vi "Open Backpressure Reader.vi"(8 "error in (no error)":errorcluster, 11 "CIPC Backpressure Names":T1) -> (0 "error out":errorcluster, 3 "CIPC BP References":T2)   [LabVIEW 2021, in "CIF_NI_CIPC.lvlib"]
uses:
  CIF_NI_CIPC.lvlib
  TypeDefs/Backpressure References.ctl
  TypeDefs/Backpressure Names.ctl
  SubVIs/Check Error.vi
  SubVIs/Get dll Path.vi
  <vilib>/Utility/error.llb/Trim Whitespace.vi
  <vilib>/Utility/error.llb/Error Cluster From Error Code.vi
  TypeDefs/Read Position.ctl
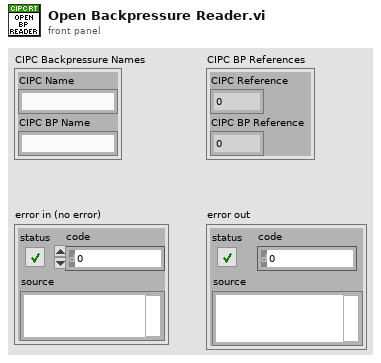
[diagram p1: front panel]
types:
  T1 = typedef "CIF_NI_CIPC.lvlib/Backpressure Names.ctl" = cluster{"CIPC Name":string, "CIPC BP Name":string}
  T2 = typedef "CIF_NI_CIPC.lvlib/Backpressure References.ctl" = cluster{"CIPC Reference":u64, "CIPC BP Reference":u64}
  T3 = typedef "CIF_NI_CIPC.lvlib/Read Position.ctl" = enum16{"Next", "Newest", "Oldest", "Next Available", "Absolute"}
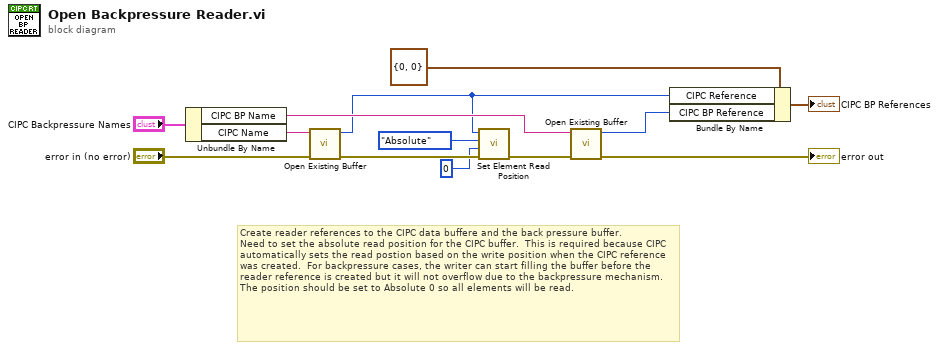
[diagram p0: block diagram]
diagram:
  # "Create reader references to the CIPC data buffere and the back pressure buffer.\nNeed to set the absolute read position for the CIPC buffer.  This is required because CIPC automatically sets the read postion based on the write position when the CIPC reference was created.  For backpressure cases, the writer can start filling the buffer before the reader reference is created but it will not overflow due to the backpressure mechanism. \nThe position should be set to Absolute 0 so all elements will be read."
  n1 = Unbundle By Name("CIPC Backpressure Names") -> ("CIPC BP Name"=w10:string, "CIPC Name"=w12:string)
  n2 = call "Open Existing Buffer.vi"("error in (no error)"="error in (no error)", "buffer_name"=w12) -> ("error out"=w3:errorcluster, "CIPC Reference"=w4:u64)  [unwired: 8 in]
  n3 = call "Set Element Read Position.vi"("error in (no error)"=w3, "Element Index Offset"=0, "Read Position"=Read_Position."Absolute", "CIPC Reference"=w4) -> ("error out"=w6:errorcluster)  [unwired: 7 in]
  n4 = call "Open Existing Buffer.vi"("error in (no error)"=w6, "buffer_name"=w10) -> ("error out"=→"error out":errorcluster, "CIPC Reference"=w7:u64)  [unwired: 8 in]
  n5 = Bundle By Name(cluster=T2 {"CIPC Reference"=0, "CIPC BP Reference"=0} ("CIPC BP References"), "CIPC Reference"=w4, "CIPC BP Reference"=w7) -> (→"CIPC BP References":T2)
